vi "containerwindow.vi"   [LabVIEW 2009]
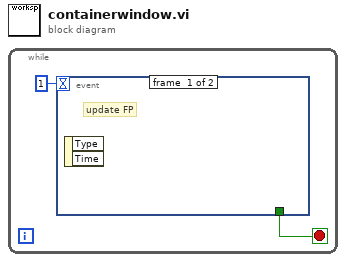
[diagram p0: block diagram]
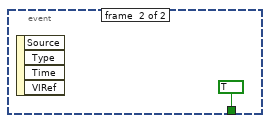
[diagram p2: hidden frame]
diagram:
  n1 = while {
    stop <- w2 stop-if-true
    n2 = event shown="[1] Panel Close" {
      selector: _ -> [_ _]
      dyn-events: _ -> [_ _]
      timeout: 1 -> [_ _]
      tunnel: [_ TRUE] -> w2
      event #0 {
        # "update FP"
        n3 = event-data() -> ()  [unwired: 3 out]
      }
      event #1 {
        n4 = event-data() -> ()  [unwired: 5 out]
      }
    }
  }
